vi "v2.vi"   [LabVIEW 2023]
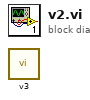
[diagram p0: block diagram]
diagram:
  n1 = call "v3.vi"() -> ()  [unwired: 12 in]
